vi "(Sub_VI)_Control_tabs_AOsignal_generation.vi"(2 "Laser Pulse Frequency (Hz)":dbl=20.0, 3 "AO Sampling Freq (KHz)":dbl=20.0, 4 "Galvo":T2={"Moving Period(ms)"=3.0, "xArray"=[1.0], "yArray"=[2.0]}, 5 "Desired Signal Param":T1={"#Up Steps"=3, "#Down Steps"=4, "Step Period(sec)"=20.0, "Min Value"=0.1, "Max Value"=0.5, "Sample Rate (Hz) = Bscan"=100.0, "Length of Desired flow in Sec]"=300.0}) -> (0 "output array of [Sti.xGalvo, Sti.yGalvo]":dbl[][](graph), 1 "Desired flow signal":dbl[](graph))   [LabVIEW 2012]
uses:
  <vilib>/Utility/error.llb/DialogType.ctl
panel:
  # "Stimulation galvo AO signal generation (for the control tabs)\nDesired hemodynamic signal generation (only for the control tabs)"
  # "Laser Pulse Frequency is used for Galvo movements If there are multiple stimulation sites then the stim galvo moves to a different location at each laser pulse.\nFor the code is designed for one stimulation spot. But the variable needs to be set properly inorder for the code to run properly"
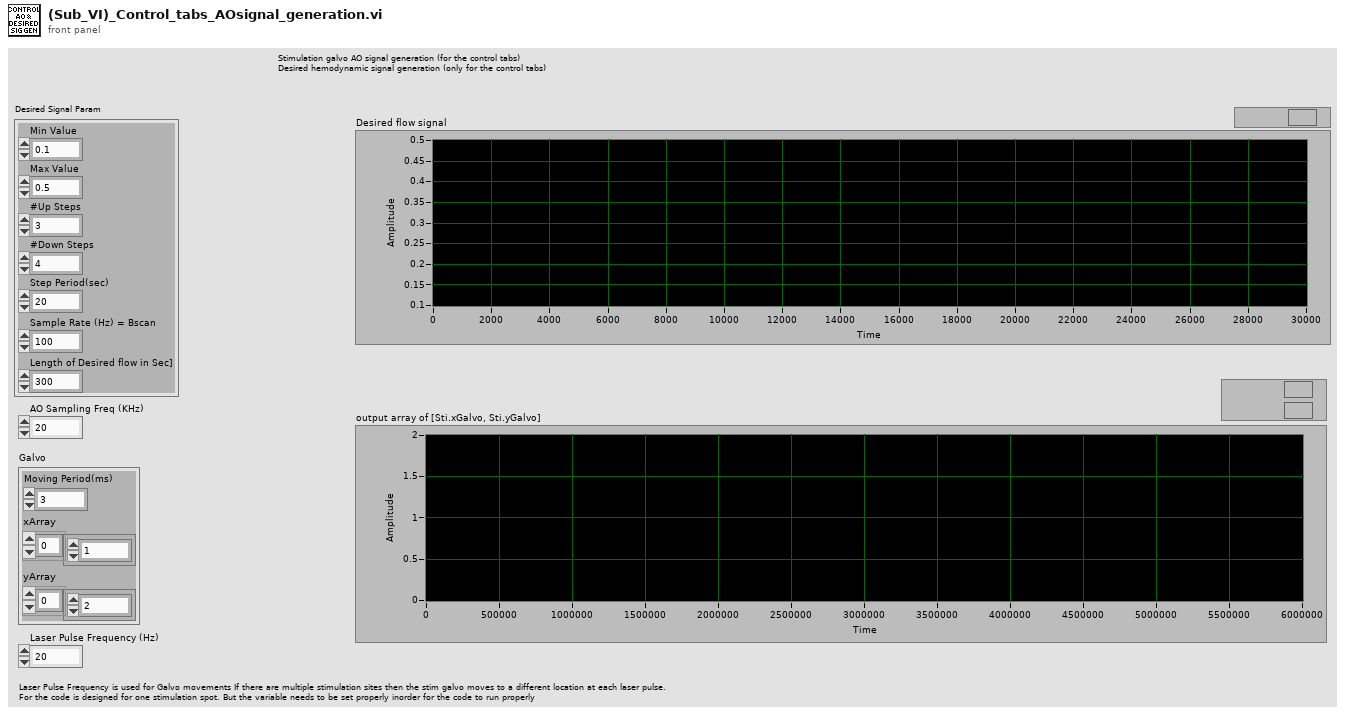
[diagram p1: front panel]
types:
  T1 = cluster{"#Up Steps":i32, "#Down Steps":i32, "Step Period(sec)":dbl, "Min Value":dbl, "Max Value":dbl, "Sample Rate (Hz) = Bscan":dbl, "Length of Desired flow in Sec]":dbl}
  T2 = cluster{"Moving Period(ms)":dbl, "xArray":dbl[], "yArray":dbl[]}
  T3 = typedef "DialogType.ctl" = u16
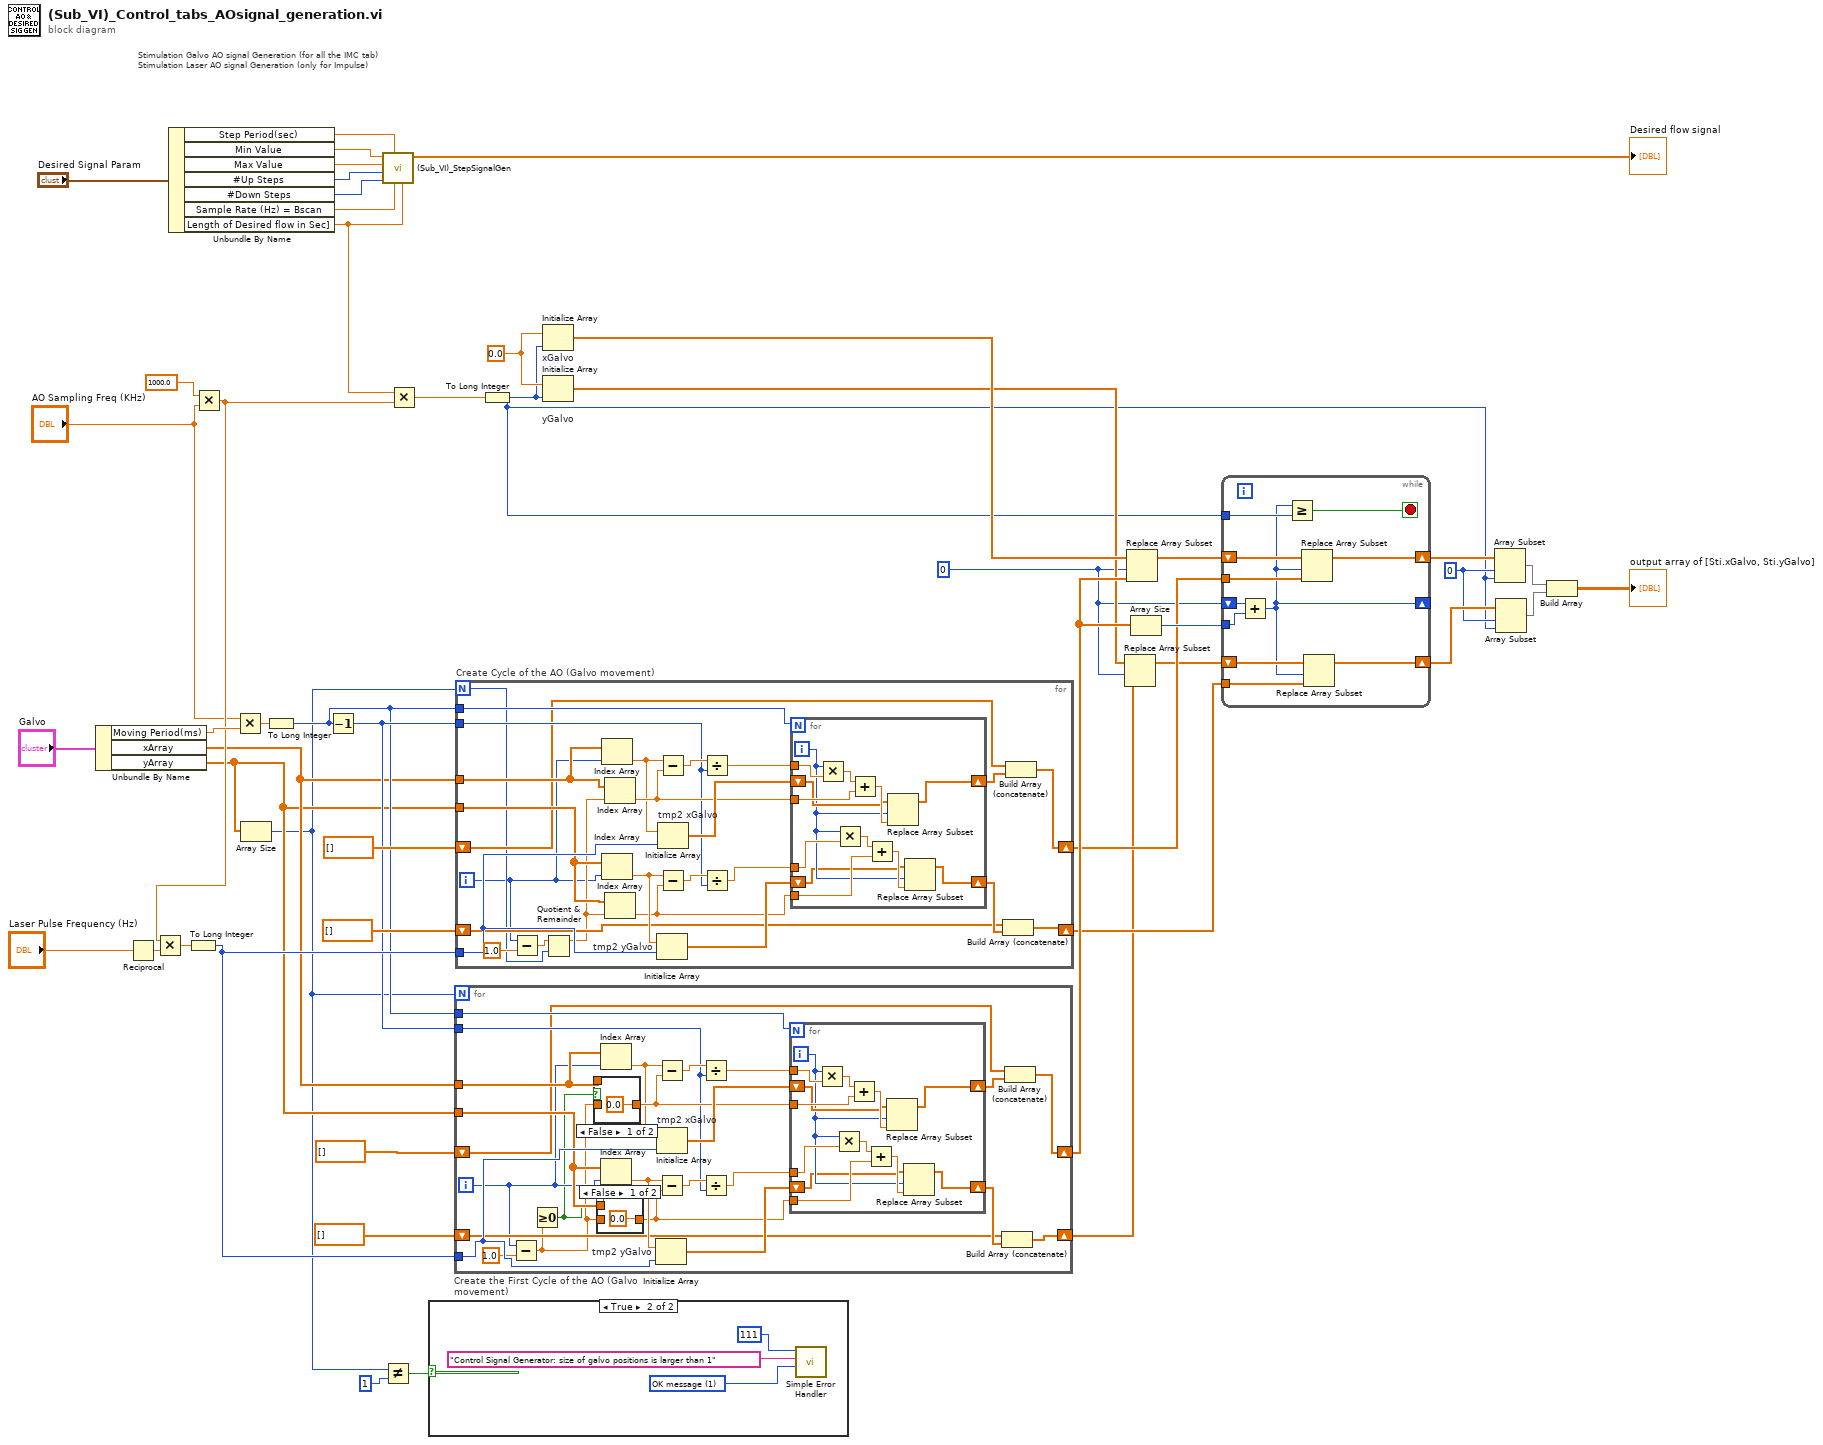
[diagram p0: block diagram]
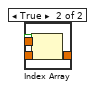
[diagram p3: hidden frame]
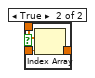
[diagram p4: hidden frame]
diagram:
  w5 = 0 ("index")
  w11 = 0
  w48 = 0.0 ("element")
  # "Stimulation Galvo AO signal Generation (for all the IMC tab)\nStimulation Laser AO signal Generation (only for Impulse)"
  n1 = Unbundle By Name("Galvo") -> ("Moving Period(ms)"=w47:dbl, "xArray"=w25:dbl[], "yArray"=w24:dbl[])
  n2 = Reciprocal(x="Laser Pulse Frequency (Hz)") -> (1/x=w45:dbl)
  n3 = Unbundle By Name("Desired Signal Param") -> ("Step Period(sec)"=w21:dbl, "Min Value"=w20:dbl, "Max Value"=w19:dbl, "#Up Steps"=w18:i32, "#Down Steps"=w17:i32, "Sample Rate (Hz) = Bscan"=w16:dbl, "Length of Desired flow in Sec]"=w10:dbl)
  n4 = Multiply(x=1000.0 ("y"), y="AO Sampling Freq (KHz)") -> (x*y=w28:dbl)
  n5 = Multiply(x=w28, y=w45) -> (x*y=w44:dbl)
  n6 = To Long Integer(number=w44) -> (32bit integer=w41:i32)
  n7 = Multiply(x="AO Sampling Freq (KHz)", y=w47) -> (x*y=w46:dbl)
  n8 = Array Size(array=w24) -> (size(s)=w13:i32)
  n9 = To Long Integer(number=w46) -> (32bit integer=w27:i32)
  n10 = Decrement(x=w27) -> (x-1=w40:i32)
  n11 = call "(Sub_VI)_StepSignalGen.vi"("Length of Desired flow (Sec)"=w10, "Sample Rate (Hz) = Bscan"=w16, "Step Period(s)"=w21, "#Down Steps"=w17, "#Up Steps"=w18, "Max Value"=w19, "Min Value"=w20) -> ("Waveform Graph"=→"Desired flow signal":dbl[])  [unwired: 4 in]
  n12 = Not Equal?(x=w13, y=1) -> (x != y?=w14:bool)
  n13 = Multiply(x=w10, y=w28) -> (x*y=w4:dbl)
  n14 = case shown="True" w14 {
    frame False {
    }
    frame True {
      w50 = T3 1 items=["no dialog", "OK message", "continue or stop message", "OK message + warnings", "continue/stop + warnings"] ("type of dialog (OK msg:1)")
      n15 = call <vilib>:"Simple Error Handler.vi"("error code (no error:0)"=111, "error source (\" \")"="Control Signal Generator: size of galvo positions is larger than 1" ("error source (\" \")"), "type of dialog (OK msg:1)"=w50) -> ()  [unwired: 2 in, 5 out]
    }
  }
  n16 = for "Create the First Cycle of the AO (Galvo movement)" {
    N: w13 -> [_]
    tunnel: w27 -> [w77]
    tunnel: w41 -> [w76]
    tunnel: w25 -> [w75]
    tunnel: w24 -> [w68]
    tunnel: w40 -> [w66]
    shift-right: [w60] -> w35
    shift-left: dbl[] [] -> [w62]
    shift-right: [w57] -> w29
    shift-left: dbl[] [] -> [w58]
    i -> [w55]
    n17 = Subtract(x=w55, y=1.0) -> (x-y=w54:dbl)
    n18 = Greater Or Equal To 0?(x=w54) -> (x >= 0?=w53:bool)
    n19 = case shown="False" w53 {
      tunnel: w75 -> [_ w85]
      tunnel: [0.0 w84] -> w71
      tunnel: w54 -> [_ w83]
      frame False {
      }
      frame True {
        n20 = Index Array(array=w85, index=w83) -> (element=w84:dbl)
      }
    }
    n21 = case shown="False" w53 {
      tunnel: w68 -> [_ w81]
      tunnel: [0.0 w80] -> w63
      tunnel: w54 -> [_ w79]
      frame False {
      }
      frame True {
        n22 = Index Array(array=w81, index=w79) -> (element=w80:dbl)
      }
    }
    n23 = Index Array(array=w75, index=w55) -> (element=w70:dbl)
    n24 = Index Array(array=w68, index=w55) -> (element=w65:dbl)
    n25 = Initialize Array "tmp2 yGalvo"(w65, w76) -> (w64:dbl[])
    n26 = Subtract(x=w70, y=w71) -> (x-y=w74:dbl)
    n27 = Initialize Array "tmp2 xGalvo"(w70, w76) -> (w72:dbl[])
    n28 = Subtract(x=w65, y=w63) -> (x-y=w69:dbl)
    n29 = Divide(x=w74, y=w66) -> (x/y=w73:dbl)
    n30 = Divide(x=w69, y=w66) -> (x/y=w67:dbl)
    n31 = for {
      N: w77 -> [_]
      tunnel: w73 -> [w96]
      shift-right: [w93] -> w61
      shift-left: w72 -> [w94]
      tunnel: w71 -> [w98]
      tunnel: w67 -> [w89]
      shift-right: [w90] -> w59
      shift-left: w64 -> [w86]
      tunnel: w63 -> [w88]
      i -> [w87]
      n32 = Multiply(x=w87, y=w96) -> (x*y=w97:dbl)
      n33 = Multiply(x=w87, y=w89) -> (x*y=w92:dbl)
      n34 = Add(x=w97, y=w98) -> (x+y=w95:dbl)
      n35 = Add(x=w92, y=w88) -> (x+y=w91:dbl)
      n36 = Replace Array Subset(array=w94, new element=w95, index=w87) -> (w93:dbl[])
      n37 = Replace Array Subset(array=w86, new element=w91, index=w87) -> (w90:dbl[])
    }
    n38 = Build Array (concatenate)(w58, w59) -> (w57:dbl[])
    n39 = Build Array (concatenate)(w62, w61) -> (w60:dbl[])
  }
  n40 = for "Create Cycle of the AO (Galvo movement)" {
    N: w13 -> [w101]
    tunnel: w27 -> [w124]
    tunnel: w41 -> [w123]
    tunnel: w25 -> [w122]
    tunnel: w24 -> [w115]
    tunnel: w40 -> [w113]
    shift-right: [w107] -> w33
    shift-left: dbl[] [] -> [w109]
    shift-right: [w104] -> w30
    shift-left: dbl[] [] -> [w105]
    i -> [w99]
    n41 = Subtract(x=w99, y=1.0) -> (x-y=w102:dbl)
    n42 = Quotient & Remainder(x=w102, y=w101) -> (x-y*floor(x/y)=w100:dbl)  [unwired: 1 out]
    n43 = Index Array(array=w122, index=w99) -> (element=w117:dbl)
    n44 = Index Array(array=w115, index=w99) -> (element=w112:dbl)
    n45 = Index Array(array=w122, index=w100) -> (element=w118:dbl)
    n46 = Index Array(array=w115, index=w100) -> (element=w110:dbl)
    n47 = Initialize Array "tmp2 yGalvo"(w112, w123) -> (w111:dbl[])
    n48 = Subtract(x=w117, y=w118) -> (x-y=w121:dbl)
    n49 = Initialize Array "tmp2 xGalvo"(w117, w123) -> (w119:dbl[])
    n50 = Subtract(x=w112, y=w110) -> (x-y=w116:dbl)
    n51 = Divide(x=w121, y=w113) -> (x/y=w120:dbl)
    n52 = Divide(x=w116, y=w113) -> (x/y=w114:dbl)
    n53 = for {
      N: w124 -> [_]
      tunnel: w120 -> [w135]
      shift-right: [w132] -> w108
      shift-left: w119 -> [w133]
      tunnel: w118 -> [w137]
      tunnel: w114 -> [w128]
      shift-right: [w129] -> w106
      shift-left: w111 -> [w125]
      tunnel: w110 -> [w127]
      i -> [w126]
      n54 = Multiply(x=w126, y=w135) -> (x*y=w136:dbl)
      n55 = Multiply(x=w126, y=w128) -> (x*y=w131:dbl)
      n56 = Add(x=w136, y=w137) -> (x+y=w134:dbl)
      n57 = Add(x=w131, y=w127) -> (x+y=w130:dbl)
      n58 = Replace Array Subset(array=w133, new element=w134, index=w126) -> (w132:dbl[])
      n59 = Replace Array Subset(array=w125, new element=w130, index=w126) -> (w129:dbl[])
    }
    n60 = Build Array (concatenate)(w105, w106) -> (w104:dbl[])
    n61 = Build Array (concatenate)(w109, w108) -> (w107:dbl[])
  }
  n62 = To Long Integer(number=w4) -> (32bit integer=w1:i32)
  n63 = Initialize Array "xGalvo"(w48, w1) -> (w37:dbl[])
  n64 = Initialize Array "yGalvo"(w48, w1) -> (w32:dbl[])
  n65 = Replace Array Subset(array=w32, new element=w29, index=w11) -> (w31:dbl[])
  n66 = Replace Array Subset(array=w37, new element=w35, index=w11) -> (w36:dbl[])
  n67 = Array Size(array=w35) -> (size(s)=w34:i32)
  n68 = while {
    shift-right: [w142] -> w9
    shift-left: w36 -> [w146]
    tunnel: w34 -> [w144]
    tunnel: w1 -> [w148]
    tunnel: w33 -> [w143]
    shift-right: [w139] -> _
    shift-left: w11 -> [w145]
    shift-right: [w140] -> w7
    shift-left: w31 -> [w141]
    tunnel: w30 -> [w138]
    stop <- w147 stop-if-true
    n69 = Add(x=w145, y=w144) -> (x+y=w139:i32)
    n70 = Greater Or Equal?(x=w139, y=w148) -> (x >= y?=w147:bool)
    n71 = Replace Array Subset(array=w146, new element=w143, index=w139) -> (w142:dbl[])
    n72 = Replace Array Subset(array=w141, new element=w138, index=w139) -> (w140:dbl[])
  }
  n73 = Array Subset(array=w9, index=w5, length=w1) -> (w8:dbl[])
  n74 = Array Subset(array=w7, index=w5, length=w1) -> (w6:dbl[])
  n75 = Build Array(w8, w6) -> (→"output array of [Sti.xGalvo, Sti.yGalvo]":dbl[][])
